vi "GetPower.vi"(8 "error in (no error)":errorcluster, 10 "Label":string, 11 "Laser_Oxxius in":refnum<class "Laser_Oxxius.lvclass">) -> (0 "error out":errorcluster, 2 "Value":dbl format="%#_13g", 3 "Laser_Oxxius out":refnum<class "Laser_Oxxius.lvclass">)   [LabVIEW 2020, in "Laser_Oxxius.lvlib" / "Laser_Oxxius.lvclass"]
uses:
  Laser_Oxxius.lvclass
  Laser_Oxxius.lvclass/Laser_Oxxius.ctl
  D:/Daguan/Development/MMicroscopyAF/Model/Real Hardware/Laser_Oxxius/Laser_Oxxius/Dependency/Oxxius_Boxx.dll
  Dependency/Oxxius_Boxx.dll
  Laser Oxxius Controller Messages/Update Power Msg/Update Power Msg.lvclass/Update Power Msg.ctl
  <vilib>/ActorFramework/Message Enqueuer/Message Enqueuer.lvclass/Message Enqueuer.ctl
  <vilib>/ActorFramework/Message Enqueuer/Enqueue.vi
  Laser Oxxius Controller Messages/Update Power Msg/Update Power Msg.lvclass
  C:/Program Files/National Instruments/LabVIEW 2020/vi.lib/ActorFramework/Message/Message.lvclass
  <vilib>/ActorFramework/Message Priority Queue/Priority Enqueue.vi
  HAL Layer/Component/Laser/Laser/Laser.lvclass
panel:
  in  "event data":cluster{"Label":string, "Value":dbl}
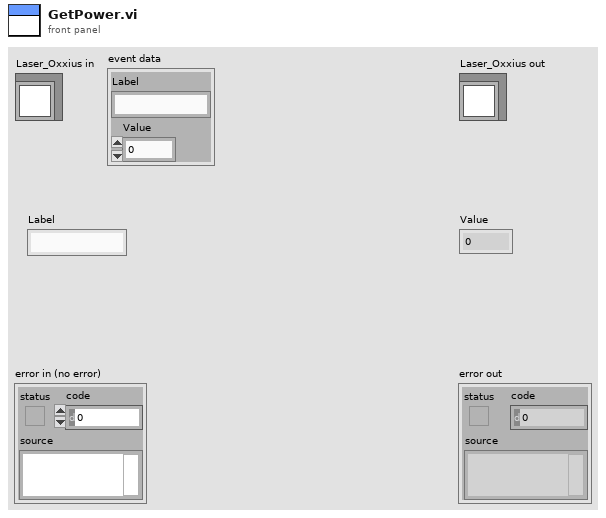
[diagram p1: front panel]
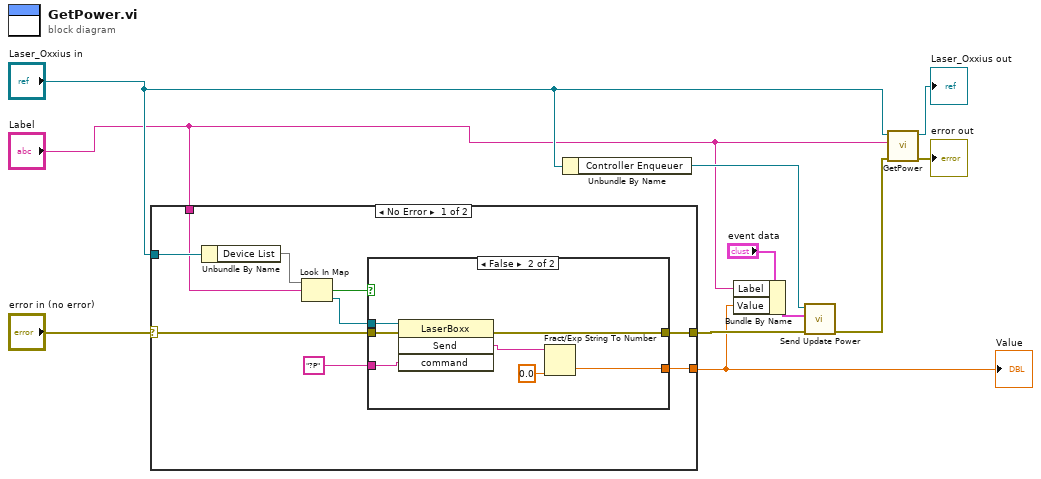
[diagram p0: block diagram]
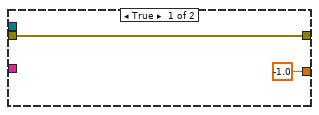
[diagram p2: hidden frame]
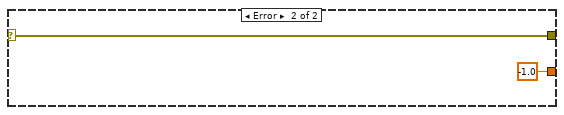
[diagram p3: hidden frame]
diagram:
  n1 = case shown="No Error" "error in (no error)" {
    selector: "error in (no error)" -> [w20 w31]
    tunnel: "Laser_Oxxius in" -> [w19 _]
    tunnel: [w15 w31] -> w7
    tunnel: "Label" -> [w17 _]
    tunnel: [w12 -1.0] -> w1
    frame No Error {
      n2 = Unbundle By Name(w19) -> ("Device List"=w18:map{string, refnum<k24>})
      n3 = Look In Map(map=w18, key=w17) -> (key not found?=w14:bool, value=w16:refnum<k24>)  [unwired: 1 in]
      n4 = case shown="False" w14 {
        tunnel: w20 -> [w22 w29]
        tunnel: w16 -> [_ w28]
        tunnel: [w22 w27] -> w15
        tunnel: "?P" ("command") -> [_ w26]
        tunnel: [-1.0 w23] -> w12
        frame True {
        }
        frame False {
          n5 = invoke class="LaserBoxx" method="Send"(reference=w28, error in=w29, "command"=w26) -> (error out=w27:errorcluster, "Send"=w24:string)  [unwired: 1 in, 2 out]
          n6 = Fract/Exp String To Number(string=w24, default (0 dbl)=0.0 ("default (0 DBL)")) -> (number=w23:dbl)  [unwired: 2 in, 1 out]
        }
      }
    }
    frame Error {
    }
  }
  "Value" <- w1
  n7 = Unbundle By Name("Laser_Oxxius in") -> ("Controller Enqueuer"=w5:refnum<class "Message Enqueuer.lvclass">)
  n8 = Bundle By Name(cluster="event data", "Label"="Label", "Value"=w1) -> (w3:cluster{"Label":string, "Value":dbl})
  n9 = call "Send Update Power.vi"("error in (no error)"=w7, "event data"=w3, "Message Enqueuer"=w5) -> ("error out"=w6:errorcluster)  [unwired: 7 in, 1 out]
  n10 = call-parent "GetPower.vi"("error in (no error)"=w6, "Label"="Label", "Laser in"="Laser_Oxxius in") -> ("error out"=→"error out":errorcluster, "Laser out"=→"Laser_Oxxius out":refnum<class "Laser_Oxxius.lvclass">)  [unwired: 6 in, 1 out]
